vi "Get Angle.vi"(4 "Axis":T1, 8 "error in (no error)":errorcluster, 11 "instrument.PPMS2 in":refnum<class "instrument.PPMS2.lvclass">) -> (0 "error out":errorcluster, 1 "Status":variant, 2 "Angle (°)":dbl, 3 "instrument.PPMS2 out":refnum<class "instrument.PPMS2.lvclass">)   [LabVIEW 2016, in "instrument.PPMS2.lvclass"]
uses:
  instrument.PPMS2.lvclass
  <userlib>/LevyLab/Levylab Instruments/Instrument Types/Cryostat/Typedefs/Rotator Axis--Enum.ctl
  Typedefs/Commands-enum.ctl
  <userlib>/LevyLab/Levylab Instruments/Instrument Types/Cryostat/Instrument.Cryostat.lvclass
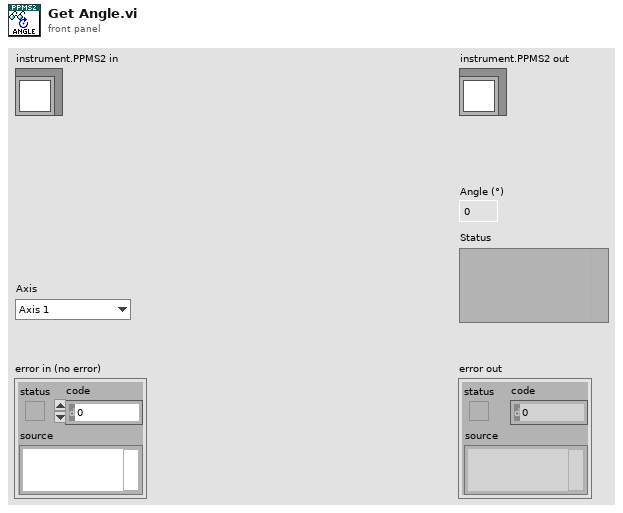
[diagram p1: front panel]
types:
  T1 = typedef "Instrument.Cryostat.lvclass/Rotator Axis--Enum.ctl" = enum16{"Axis 1", "Axis 2"}
  T2 = typedef "instrument.PPMS2.lvclass/Commands-enum.ctl" = enum16{"Get Magnet Field", "Get Helium Level", "Get Temperature", "Get Angle", "Set Magnet Field", "Set Temperature", "Set Angle", "getAll"}
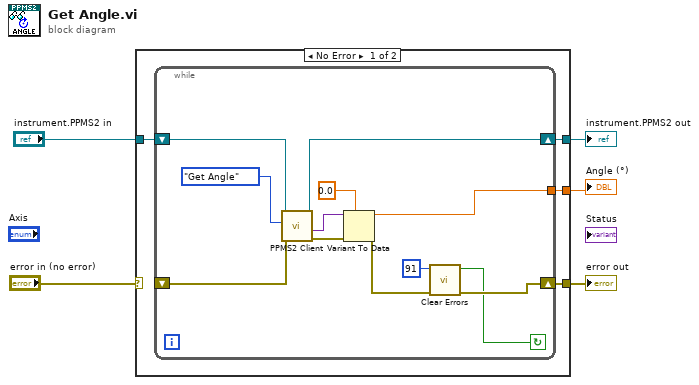
[diagram p0: block diagram]
diagram:
  n1 = case shown="No Error" "error in (no error)" {
    selector: "error in (no error)" -> [_ w23]
    tunnel: [w6 _] -> w5
    tunnel: [w9 w23] -> w4
    tunnel: "instrument.PPMS2 in" -> [w7 w22]
    tunnel: [w8 w22] -> w1
    frame No Error {
      n2 = while {
        tunnel: [w14] -> w6
        shift-right: [w13] -> w9
        shift-left: _ -> [w20]
        shift-right: [w19] -> w8
        shift-left: w7 -> [w18]
        stop <- w11 continue-if-true
        n3 = call "PPMS2 Client.vi"("error in (no error)"=w20, "Command"=Commands-enum."Get Angle" ("Enum"), "instrument.PPMS2 in"=w18) -> ("error out"=w16:errorcluster, "Data out"=w15:variant, "instrument.PPMS2 out"=w19:refnum<class "instrument.PPMS2.lvclass">)  [unwired: 5 in, 1 out]
        n4 = Variant To Data(error in=w16, type=0.0 ("Position (Degree)"), Variant=w15) -> (data=w14:dbl, error out=w21:errorcluster)
        n5 = call <vilib>:"Clear Errors.vi"("error in (no error)"=w21, "specific error code to clear (0: all)"=91) -> ("error out"=w13:errorcluster, "specific error cleared?"=w11:bool)  [unwired: 4 in]
      }
    }
    frame Error {
    }
  }
  "error out" <- w4
  "instrument.PPMS2 out" <- w1
  "Angle (°)" <- w5
